vi "serialPorts.vi"(8 "list?":bool=TRUE, 11 "Python version":string) -> (0 "error out":errorcluster, 1 "ports":string[](array[string]), 2 "appended path":path, 3 "Refnum out":refnum<k35>)   [LabVIEW 2022 SP3]
panel:
  out "find list":string[](array[string])
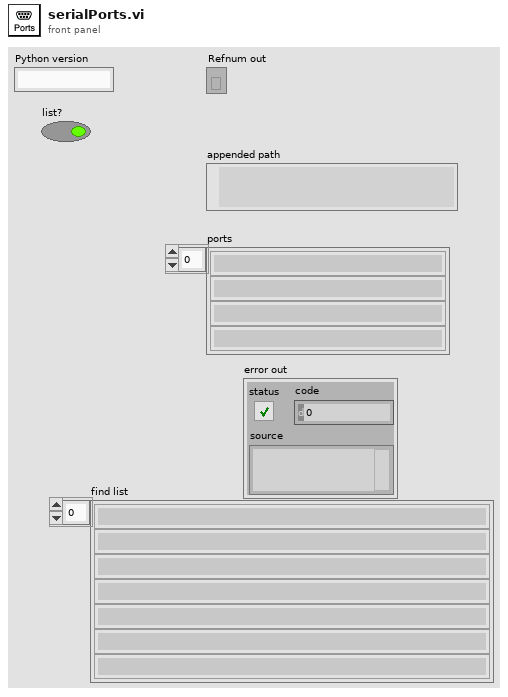
[diagram p1: front panel]
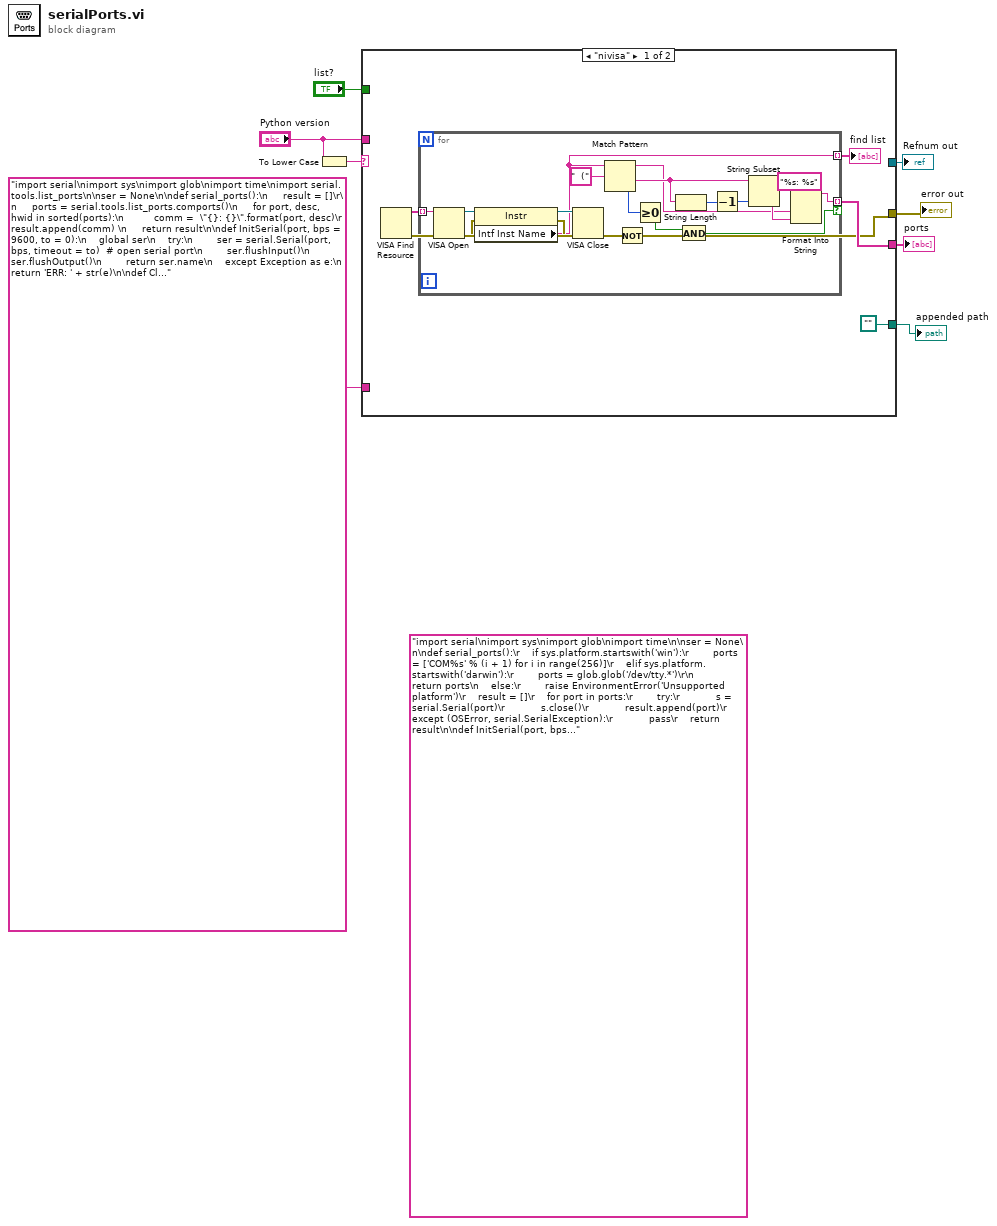
[diagram p0: block diagram]
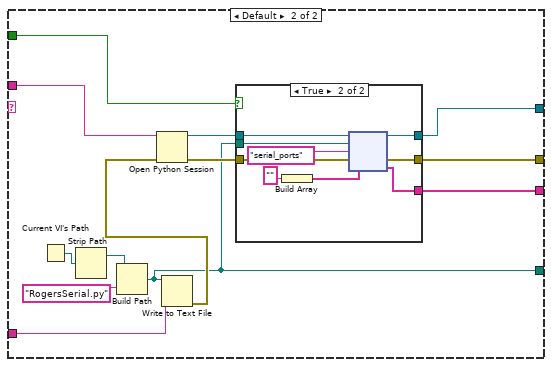
[diagram p2: hidden frame]
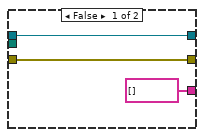
[diagram p3: hidden frame]
diagram:
  (unwired) "import serial\nimport sys\nimport glob\nimport time\n\nser = None\n\ndef serial_ports():\r    if sys.platform.startswith('win'):\r        ports = ['COM%s' % (i + 1) for i in range(256)]\r    elif sys.platform.startswith('darwin'):\r        ports = glob.glob('/dev/tty.*')\r\n        return ports\n    else:\r        raise EnvironmentError('Unsupported platform')\r    result = []\r    for port in ports:\r        try:\r            s = serial.Serial(port)\r            s.close()\r            result.append(port)\r        except (OSError, serial.SerialException):\r            pass\r    return result\n\ndef InitSerial(port, bps = 9600, to = 0):\n    global ser\n    try:\n        ser = serial.Serial(port, bps, timeout = to)  # open serial port\n        ser.flushInput()\n        ser.flushOutput()\n        return ser.name\n    except Exception as e:\n        return 'ERR: ' + str(e)\n\ndef FlushSerial():\n    ser.flushInput()\n    ser.flushOutput()\n    return(ser.in_waiting)\n\ndef CloseSerial():\n    ser.flush()\n    ser.close()\n    return('done')\n\ndef WriteSerial(string):\n    try:\n        reply = ser.write(string.encode())\n        return str(reply)\n    except Exception as e:\n        return 'ERR: ' + str(e)    \n\ndef WriteBytes(data,replyLength):\n    buffer=ser.read(ser.in_waiting)\n    reply = ser.write(bytes(data))\n    if (replyLength < 0): return []\n    return list(ser.read(replyLength))    # write bytes and get reply\n\ndef ScriptSerial(string):\n    reply = ''\n    lines = string.split('\\n')\n    for line in lines:\n        ser.write(line.encode())\n        time.sleep(1)\n        reply += ReadSerial() + '\\n'\n    return reply \n\ndef ReadSerial():\n    try:\n        reply = ''\n        if ser.in_waiting:\n            reply = ser.readline().decode()\n        return reply\n    except Exception as e:\n        return 'ERR: ' +  str(e)\n\n# note if the timeout is anything but zero it is slow"
  n1 = To Lower Case(string="Python version") -> (all lower case string=w2:string)
  n2 = case shown="\"nivisa\"" w2 {
    tunnel: [w10 w44] -> w8
    tunnel: [w11 w43] -> w7
    tunnel: "Python version" -> [_ w42]
    tunnel: "import serial\nimport sys\nimport glob\nimport time\nimport serial.tools.list_ports\n\nser = None\n\ndef serial_ports():\n     result = []\r\n     ports = serial.tools.list_ports.comports()\n     for port, desc, hwid in sorted(ports):\n          comm =  \"{}: {}\".format(port, desc)\r          result.append(comm) \n     return result\n\ndef InitSerial(port, bps = 9600, to = 0):\n    global ser\n    try:\n        ser = serial.Serial(port, bps, timeout = to)  # open serial port\n        ser.flushInput()\n        ser.flushOutput()\n        return ser.name\n    except Exception as e:\n        return 'ERR: ' + str(e)\n\ndef CloseSerial():\n    return('done')\n    try:\n        ser.flush()\n        ser.close()\n        return 'done'\n    except Exception as e:\n        return 'ERR: ' + str(e)    \n\ndef WriteSerial(string):\n    try:\n        reply = ser.write(string.encode())\n        return str(reply)\n    except Exception as e:\n        return 'ERR: ' + str(e)    \n\ndef WriteBytes(data,replyLength):\n    try:\n        buffer=ser.read(ser.in_waiting)\n        reply = ser.write(bytes(data))\n        if (replyLength < 0): return []\n        return list(ser.read(replyLength))    # write bytes and get reply\n    except Exception as e:\n        return 'ERR: ' + str(e)    \n\ndef ReadSerial():\n    try:\n        reply = ''\n        if ser.in_waiting:\n            reply = ser.readline().decode()\n        return reply\n    except Exception as e:\n        return 'ERR: ' +  str(e)\n\n# note if the timeout is anything but zero it is slow" -> [_ w39]
    tunnel: [_ w37] -> w5
    tunnel: "list?" -> [_ w34]
    tunnel: [path "" w33] -> w1
    frame "nivisa" {
      n3 = VISA Find Resource() -> (0:w10:errorcluster, 3:w12:string[])  [unwired: 3 in, 1 out]
      n4 = for {
        tunnel: w12 -> [w32] mode=indexing
        tunnel: [w24] -> w11 mode=indexing if=w17
        tunnel: [w16] -> w13 mode=indexing
        n5 = VISA Open(VISA resource name=w32) -> (VISA resource name=w23:refnum<visa-resource-name>, error out=w21:errorcluster)  [unwired: 4 in]
        n6 = property class="Instr"(reference=w23, error in=w21) -> (reference out=w31:refnum<visa-resource-name>, error out=w22:errorcluster, "Intf Inst Name"=w16:string)
        n7 = VISA Close(VISA resource name=w31, error in (no error)=w22) -> (error out=w30:errorcluster)
        n8 = Match Pattern(string=w16, regular expression="  (") -> (before substring=w14:string, after substring=w27:string, offset past match=w20:i32)  [unwired: 1 in, 1 out]
        n9 = Not(x=w30) -> (.not. x?=w19:bool)
        n10 = Greater Or Equal To 0?(x=w20) -> (x >= 0?=w18:bool)
        n11 = String Length(string=w27) -> (length=w26:i32)
        n12 = And(x=w18, y=w19) -> (x .and. y?=w17:bool)
        n13 = Decrement(x=w26) -> (x-1=w25:i32)
        n14 = String Subset(string=w27, length (rest)=w25) -> (substring=w15:string)  [unwired: 1 in]
        n15 = Format Into String(format string="%s: %s", w14, w15) -> (resulting string=w24:string)  [unwired: 2 in, 1 out]
      }
      "find list" <- w13
    }
    frame Default {
      n16 = Current VI's Path() -> (path=w40:path)
      n17 = Strip Path(path=w40) -> (stripped path=w41:path)  [unwired: 1 out]
      n18 = Build Path(base path=w41, name or relative path="RogersSerial.py") -> (appended path=w33:path)
      n19 = Write to Text File(file (use dialog)=w33, text=w39) -> (error out=w36:errorcluster)  [unwired: 2 in, 2 out]
      n20 = Open Python Session(python version=w42, 3:w36) -> (session out=w45:refnum<k35>, error out=w35:errorcluster)  [unwired: 1 in]
      n21 = case shown="True" w34 {
        tunnel: w33 -> [_ w57]
        tunnel: w45 -> [w48 w56]
        tunnel: [w47 w55] -> w44
        tunnel: [string[] [] w54] -> w43
        tunnel: [w48 w50] -> w37
        tunnel: w35 -> [w47 w49]
        frame False {
        }
        frame True {
          n22 = Build Array("" ("function name")) -> (w53:string[])
          n23 = node(w56, w57, "serial_ports" ("function name"), w49, w53) -> (w50:refnum<k35>, w55:errorcluster, w54:string[])  [unwired: 2 out]
        }
      }
    }
  }
  "Refnum out" <- w5
  "error out" <- w8
  "ports" <- w7
  "appended path" <- w1
